vi "test.vi"() -> ()   [LabVIEW 2012]
uses:
  G_SEN.vi
panel:
  out "Array 6":dbl[][](array[numeric])
  out "Array 5":dbl[](array[numeric])
  out "Array 4":i32[](array[numeric])
  out "x*y":dbl[](array[numeric])
  out "Array":dbl[][](array[numeric])
  out "XY Graph 2":cluster{"Y":dbl[], "Y":dbl[]}[](graph)
  out "Array 3":dbl[](array[numeric])
  out "Array 2":cluster{dbl[][]}[](array[cluster])
  out "error out":errorcluster
  out "XY Graph":cluster{"Y":dbl[], "Y":dbl[]}[](graph)
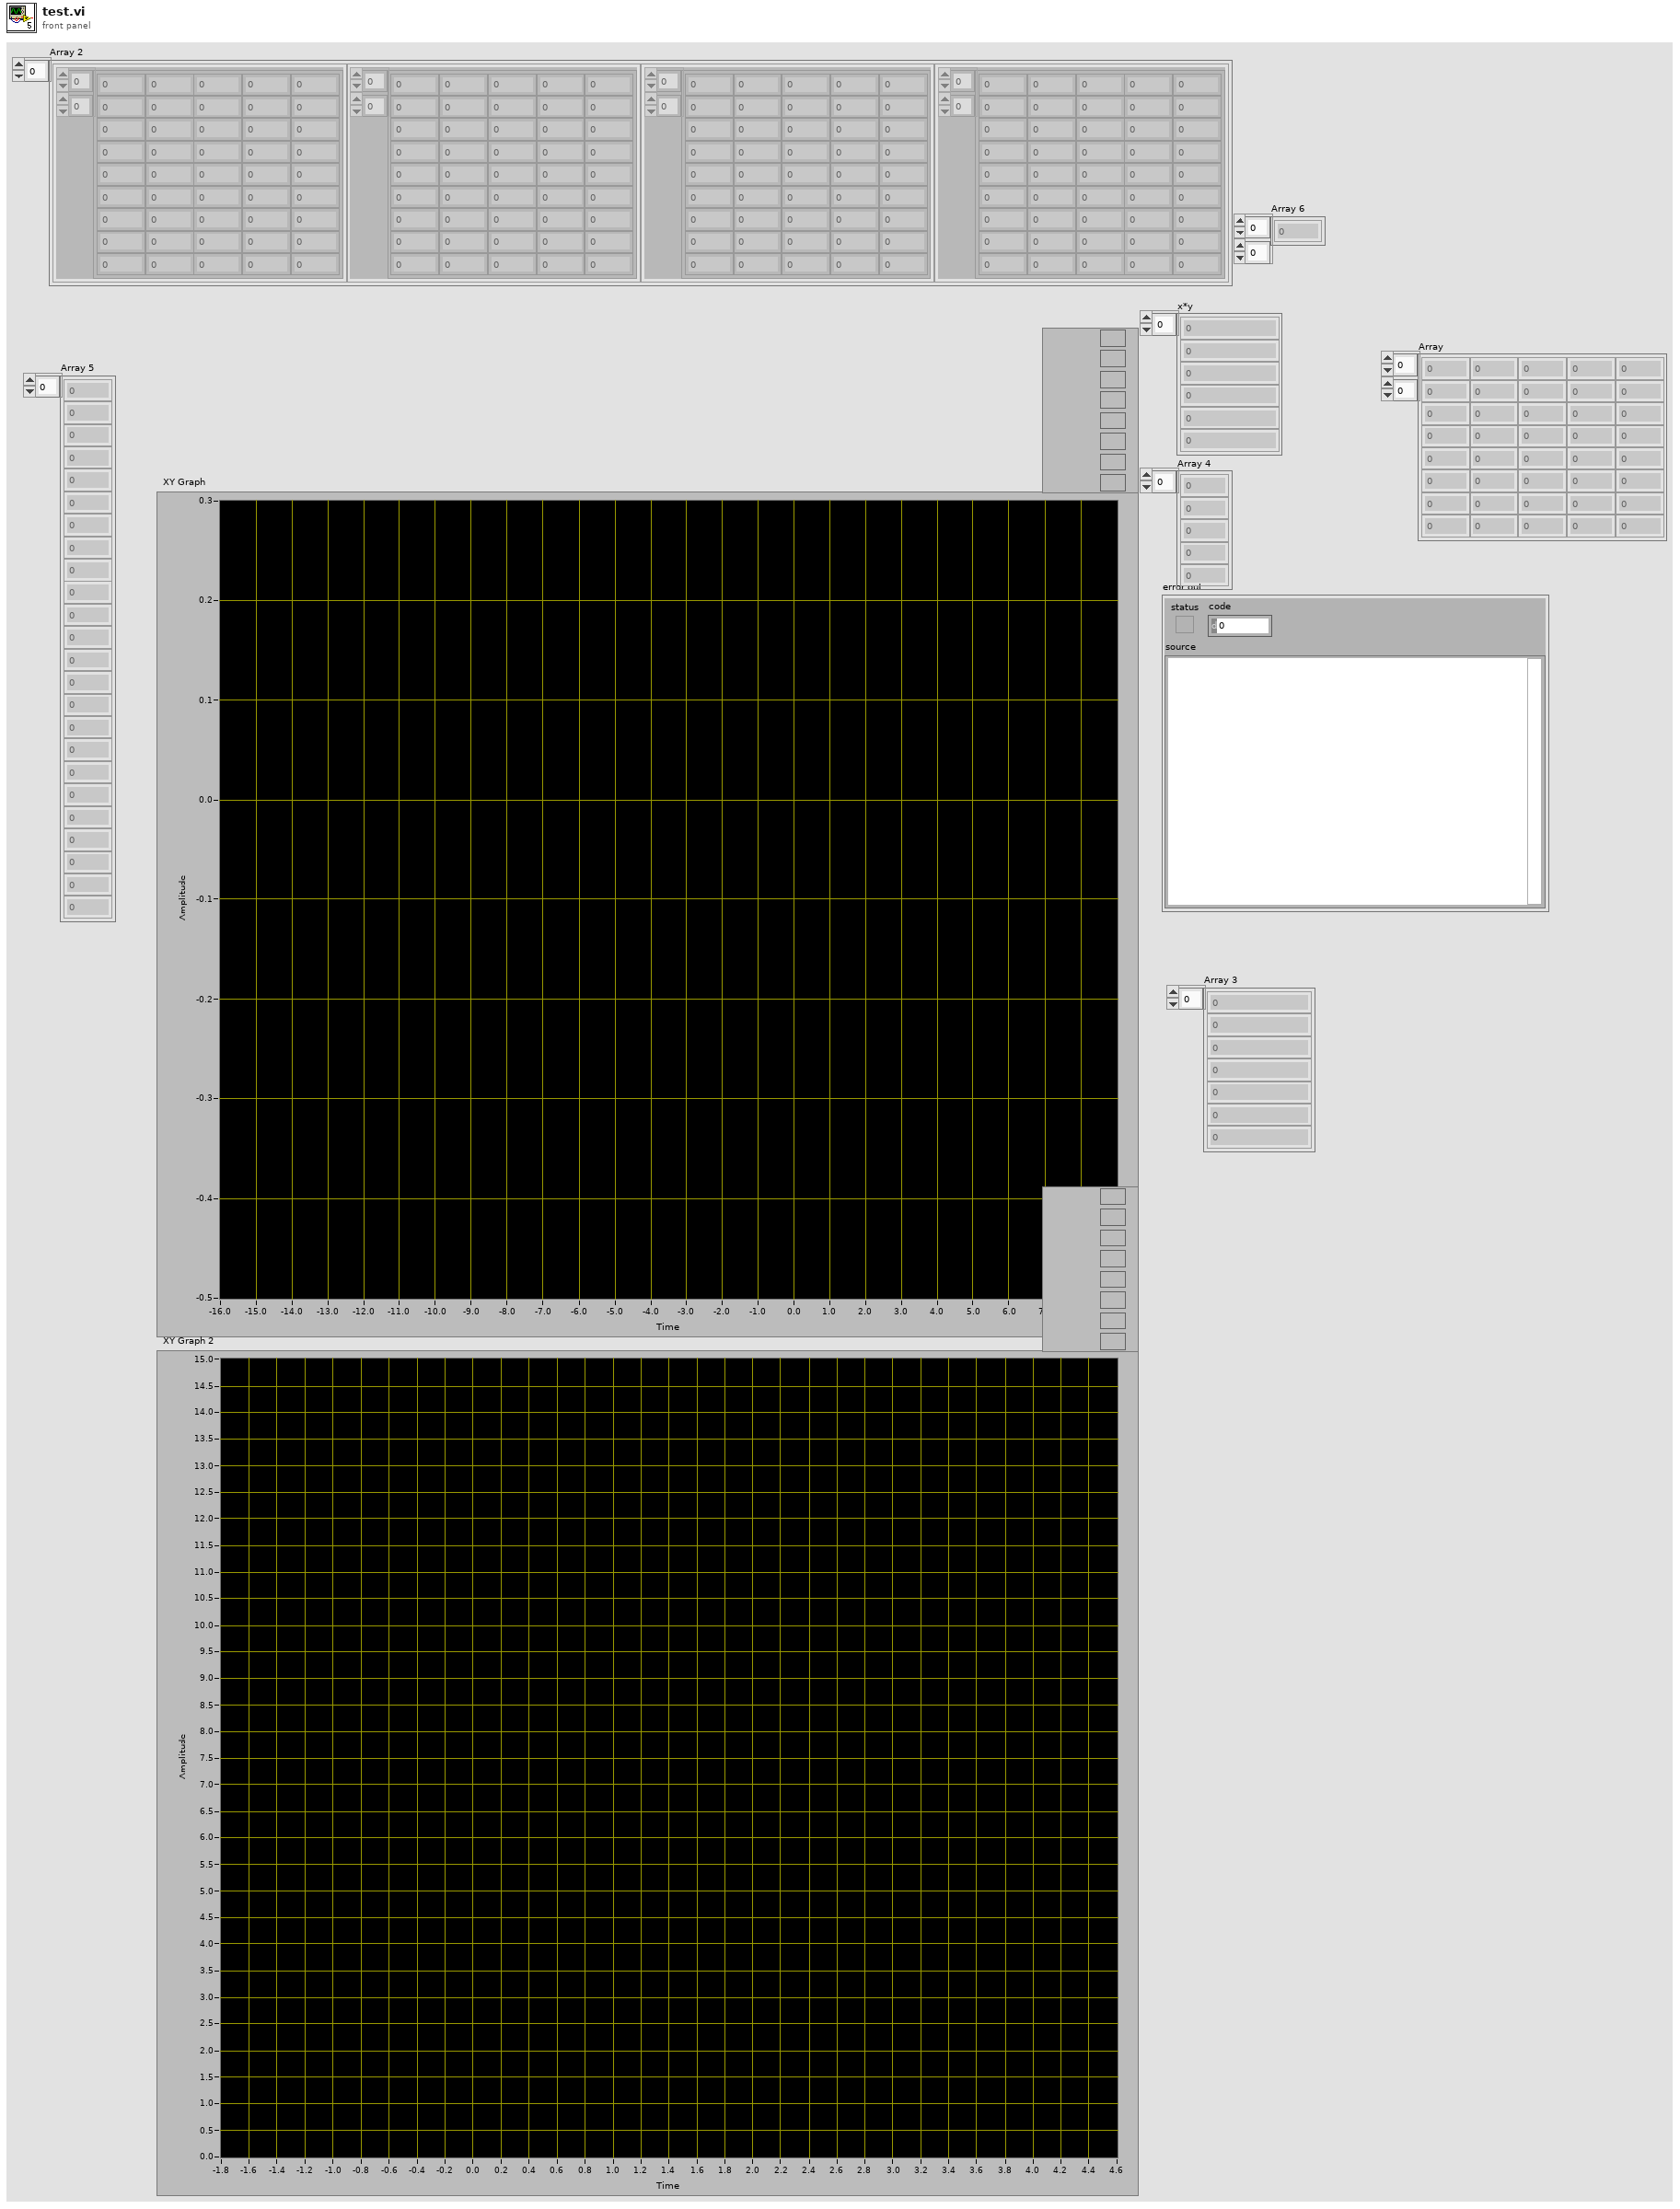
[diagram p1: front panel]
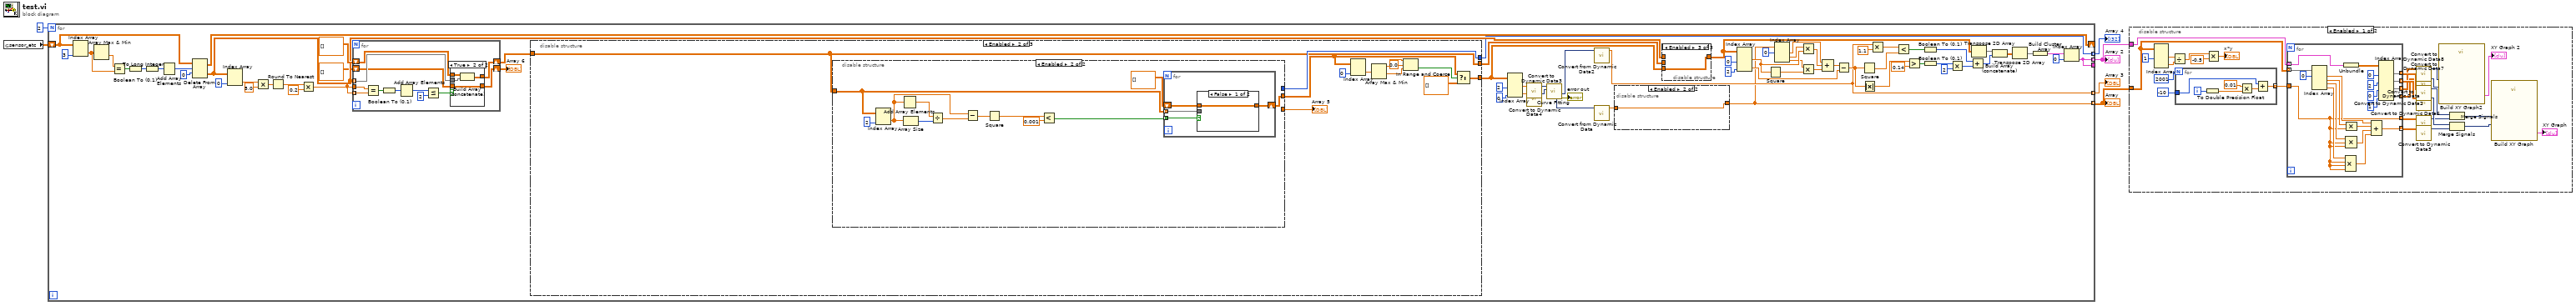
[diagram p0: block diagram]
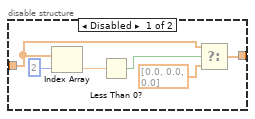
[diagram p3: hidden frame]
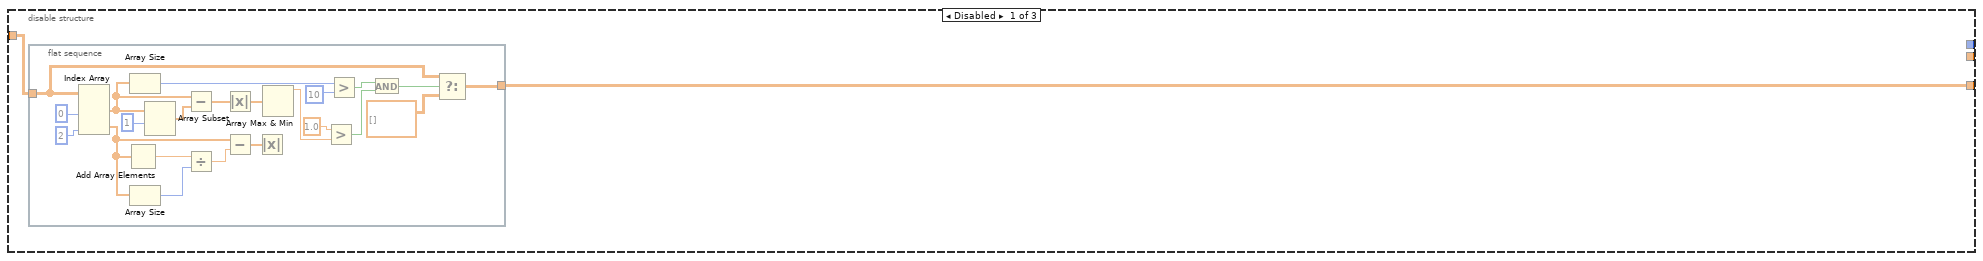
[diagram p4: hidden frame]
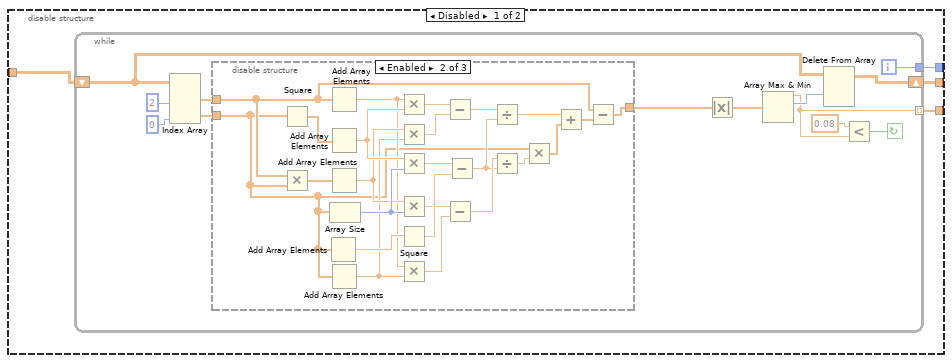
[diagram p5: hidden frame]
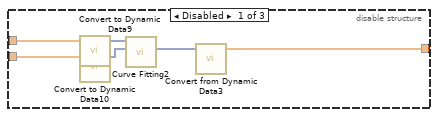
[diagram p6: hidden frame]
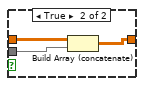
[diagram p8: hidden frame]
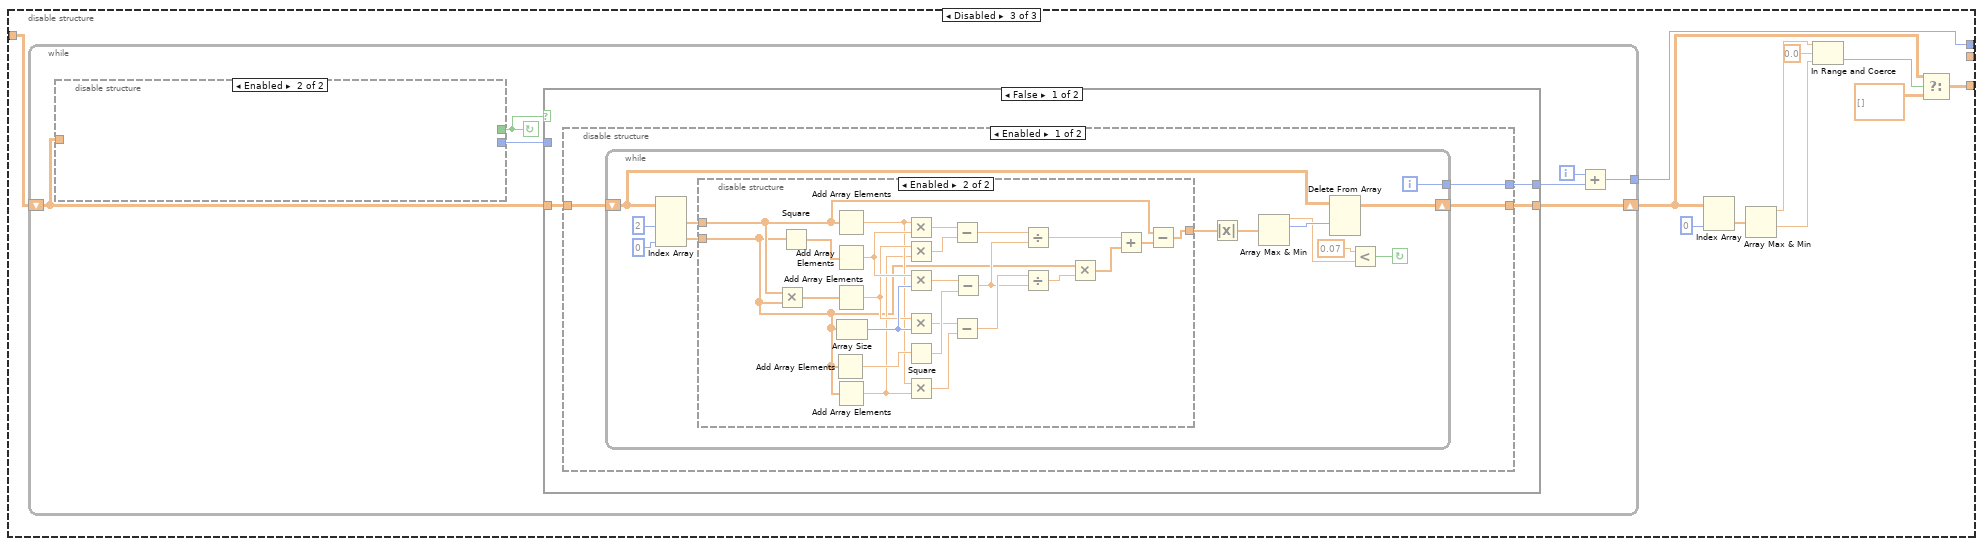
[diagram p9: hidden frame]
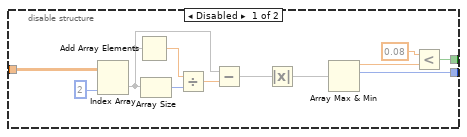
[diagram p10: hidden frame]
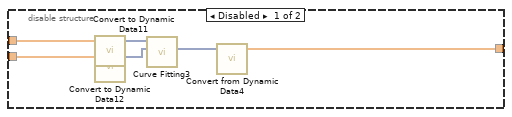
[diagram p11: hidden frame]
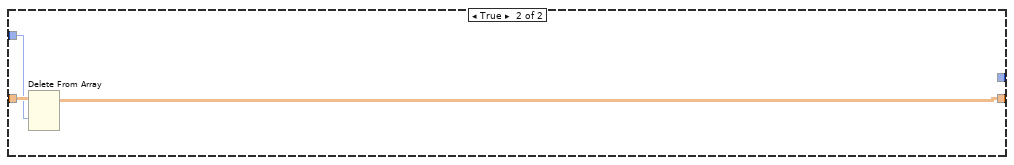
[diagram p13: hidden frame]
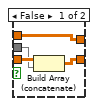
[diagram p16: hidden frame]
diagram:
  n1 = global read "G_SEN.vi" "sensor_etc"() -> (w5:dbl[][])
  n2 = for {
    N: 2 -> [_]
    shift-right: [w66] -> _
    shift-left: w5 -> [w69]
    tunnel: [w14] -> _
    tunnel: [w14] -> w3 mode=indexing
    tunnel: [w13] -> w4 mode=indexing
    tunnel: [w11] -> w2 mode=indexing
    tunnel: [w10] -> w1 mode=indexing
    n3 = Index Array(array=w69, index (col)=3 ("disabled index (col)")) -> (element=w73:dbl[])  [unwired: 1 in]
    n4 = Array Max & Min(array=w73) -> (min value=w74:dbl)  [unwired: 3 out]
    n5 = Equal?(x=w74, y=w73) -> (x = y?=w72:bool[])
    n6 = Boolean To (0,1)(Boolean=w72) -> (0, 1=w71:i16[])
    n7 = To Long Integer(number=w71) -> (32bit integer=w70:i32[])
    n8 = Add Array Elements(numeric array=w70) -> (sum=w68:i32)
    n9 = Delete From Array(array=w69, length=w68, index (row)=0) -> (deleted portion=w18:dbl[][], array with subset deleted=w66:dbl[][])  [unwired: 1 in]
    n10 = Index Array(array=w18, index (col)=0 ("disabled index (col)")) -> (element=w62:dbl[])  [unwired: 1 in]
    n11 = Multiply(x=w62, y=5.0) -> (x*y=w60:dbl[])
    n12 = Round To Nearest(number=w60) -> (nearest integer value=w59:dbl[])
    n13 = Multiply(x=w59, y=0.2) -> (x*y=w57:dbl[])
    n14 = for {
      tunnel: w57 -> [w275] mode=indexing
      tunnel: w57 -> [w283]
      shift-right: [w278] -> w16
      shift-left: dbl[][] [] -> [w279]
      tunnel: w18 -> [w280] mode=indexing
      shift-right: [w272] -> w7
      shift-left: dbl[][] [] -> [w273]
      n15 = Equal?(x=w283, y=w275) -> (x = y?=w282:bool[])
      n16 = Boolean To (0,1)(Boolean=w282) -> (0, 1=w281:i16[])
      n17 = Add Array Elements(numeric array=w281) -> (sum=w277:i16)
      n18 = Less Or Equal?(x=w277, y=i16 2) -> (x <= y?=w274:bool)
      n19 = case shown="True" w274 {
        tunnel: w280 -> [w284 w291]
        tunnel: w279 -> [w287 w290]
        tunnel: [w287 w289] -> w278
        tunnel: w273 -> [w286 w288]
        tunnel: [w285 w288] -> w272
        frame False {
          n20 = Build Array (concatenate)(w286, w284) -> (w285:dbl[][])
        }
        frame True {
          n21 = Build Array (concatenate)(w290, w291) -> (w289:dbl[][])
        }
      }
    }
    "Array 6" <- w7
    n22 = disable-structure shown="Enabled" {
      disable-tunnel: w16 -> [w84 w107 w196]
      disable-tunnel: [w83 w111 w188] -> w15
      disable-tunnel: [_ w109 w186] -> w10
      disable-tunnel: [_ w107 _] -> w9
      frame Disabled {
        n23 = flat-sequence {
          tunnel: w84 -> [w95]
          tunnel: [w94] -> w83
          frame #0 {
            n24 = Index Array(array=w95, index (col) #1=0 ("disabled index (col)"), index (col) #2=2 ("index (col)")) -> (element #1=w102:dbl[], element #2=w86:dbl[])  [unwired: 2 in]
            n25 = Add Array Elements(numeric array=w86) -> (sum=w89:dbl)
            n26 = Array Size(array=w102) -> (size(s)=w101:i32)
            n27 = Array Size(array=w86) -> (size(s)=w88:i32)
            n28 = Array Subset(array=w102, index=1) -> (w103:dbl[])  [unwired: 1 in]
            n29 = Subtract(x=w102, y=w103) -> (x-y=w106:dbl[])
            n30 = Divide(x=w89, y=w88) -> (x/y=w87:dbl)
            n31 = Absolute Value(x=w106) -> (abs(x)=w99:dbl[])
            n32 = Subtract(x=w86, y=w87) -> (x-y=w85:dbl[])
            n33 = Absolute Value(x=w85) -> ()  [unwired: 1 out]
            n34 = Array Max & Min(array=w99) -> (max value=w98:dbl)  [unwired: 3 out]
            n35 = Greater?(x=1.0, y=w98) -> (0:w91:bool)
            n36 = Greater?(x=w101, y=10) -> (0:w92:bool)
            n37 = And(x=w92, y=w91) -> (x .and. y?=w96:bool)
            n38 = Select(t=w95, s=w96, f=dbl[][] []) -> (s? t:f=w94:dbl[][])
          }
        }
      }
      frame Enabled {
        n39 = disable-structure shown="Enabled" {
          disable-tunnel: w107 -> [w122 w171]
          disable-tunnel: [w121 w166] -> w112
          disable-tunnel: [w120 _] -> w109
          disable-tunnel: [w119 _] -> w108
          frame Disabled {
            n40 = while {
              shift-right: [w130] -> w121
              shift-left: w122 -> [w131]
              tunnel: [w127] -> w120
              tunnel: [w123] -> w119 mode=indexing
              i -> [w127]
              stop <- w128 continue-if-true
              n41 = Index Array(array=w131, index (col) #1=2 ("disabled index (col)"), index (col) #2=0 ("index (col)")) -> (element #1=w135:dbl[], element #2=w124:dbl[])  [unwired: 2 in]
              n42 = disable-structure shown="Enabled" {
                disable-tunnel: w135 -> [w141 w147 _]
                disable-tunnel: [w137 w146 _] -> w126
                disable-tunnel: w124 -> [w136 w144 _]
                frame Disabled {
                  n43 = call "Convert to Dynamic Data9"("Array"=w141) -> ("Dynamic Data Type"=w139:dynamicdata)  [unwired: 3 in]
                  n44 = call "Convert to Dynamic Data10"("Array"=w136) -> ("Dynamic Data Type"=w140:dynamicdata)  [unwired: 3 in]
                  n45 = call "Curve Fitting2"("Locations"=w140, "Signals"=w139) -> ("residual"=w138:dynamicdata)  [unwired: 5 in, 4 out]
                  n46 = call "Convert from Dynamic Data3"("Dynamic Data Type"=w138) -> ("Array"=w137:dbl[])  [unwired: 3 in]
                }
                frame Enabled {
                  n47 = Square(x=w144) -> (x^2=w165:dbl[])
                  n48 = Multiply(x=w147, y=w144) -> (x*y=w161:dbl[])
                  n49 = Add Array Elements(numeric array=w144) -> (sum=w164:dbl)
                  n50 = Add Array Elements(numeric array=w147) -> (sum=w153:dbl)
                  n51 = Add Array Elements(numeric array=w165) -> (sum=w162:dbl)
                  n52 = Add Array Elements(numeric array=w161) -> (sum=w155:dbl)
                  n53 = Add Array Elements(numeric array=w144) -> (sum=w152:dbl)
                  n54 = Array Size(array=w144) -> (size(s)=w156:i32)
                  n55 = Multiply(x=w153, y=w162) -> (x*y=w159:dbl)
                  n56 = Multiply(x=w155, y=w152) -> (x*y=w160:dbl)
                  n57 = Multiply(x=w162, y=w156) -> (x*y=w157:dbl)
                  n58 = Multiply(x=w155, y=w156) -> (x*y=w154:dbl)
                  n59 = Square(x=w164) -> (x^2=w163:dbl)
                  n60 = Multiply(x=w153, y=w152) -> (x*y=w151:dbl)
                  n61 = Subtract(x=w159, y=w160) -> (x-y=w158:dbl)
                  n62 = Subtract(x=w154, y=w151) -> (x-y=w150:dbl)
                  n63 = Subtract(x=w157, y=w163) -> (x-y=w149:dbl)
                  n64 = Divide(x=w158, y=w149) -> (x/y=w145:dbl)
                  n65 = Divide(x=w150, y=w149) -> (x/y=w143:dbl)
                  n66 = Multiply(x=w144, y=w143) -> (x*y=w142:dbl[])
                  n67 = Add(x=w145, y=w142) -> (x+y=w148:dbl[])
                  n68 = Subtract(x=w147, y=w148) -> (x-y=w146:dbl[])
                }
                frame Disabled {
                }
              }
              n69 = Absolute Value(x=w126) -> (abs(x)=w125:dbl[])
              n70 = Array Max & Min(array=w125) -> (max value=w123:dbl, max index (indices)=w132:i32)  [unwired: 2 out]
              n71 = Delete From Array(array=w131, index (row)=w132) -> (array with subset deleted=w130:dbl[][])  [unwired: 2 in, 1 out]
              n72 = Less?(x=0.08, y=w123) -> (x < y?=w128:bool)
            }
          }
          frame Enabled {
            n73 = Index Array(array=w171, index (col)=2 ("disabled index (col)")) -> (element=w173:dbl[])  [unwired: 1 in]
            n74 = Add Array Elements(numeric array=w173) -> (sum=w176:dbl)
            n75 = Array Size(array=w173) -> (size(s)=w172:i32)
            n76 = Divide(x=w176, y=w172) -> (x/y=w175:dbl)
            n77 = Subtract(x=w173, y=w175) -> (x-y=w174:dbl[])
            n78 = Square(x=w174) -> (x^2=w170:dbl[])
            n79 = Less?(x=w170, y=0.001) -> (x < y?=w168:bool[])
            n80 = for {
              tunnel: w171 -> [w180] mode=indexing
              tunnel: w168 -> [w181] mode=indexing
              shift-right: [w178] -> w166
              shift-left: dbl[][] [] -> [w179]
              n81 = case shown="False" w181 {
                tunnel: w180 -> [_ w185]
                tunnel: w179 -> [w182 w184]
                tunnel: [w182 w183] -> w178
                frame False {
                }
                frame True {
                  n82 = Build Array (concatenate)(w184, w185) -> (w183:dbl[][])
                }
              }
            }
          }
        }
        "Array 5" <- w108
        n83 = Index Array(array=w112, index (col)=0 ("disabled index (col)")) -> (element=w117:dbl[])  [unwired: 1 in]
        n84 = Array Max & Min(array=w117) -> (max value=w116:dbl, min value=w115:dbl)  [unwired: 2 out]
        n85 = In Range and Coerce(upper limit=w116, x=0.0, lower limit=w115) -> (In Range?=w113:bool)  [unwired: 1 out]
        n86 = Select(t=w112, s=w113, f=dbl[][] []) -> (s? t:f=w111:dbl[][])
      }
      frame Disabled {
        n87 = while {
          shift-right: [w201] -> w189
          shift-left: w196 -> [w202]
          tunnel: [w197] -> w186
          i -> [w199]
          stop <- w203 continue-if-true
          n88 = disable-structure shown="Enabled" {
            disable-tunnel: [w207 _] -> w203
            disable-tunnel: w202 -> [w206 _]
            disable-tunnel: [w205 _] -> w200
            frame Disabled {
              n89 = Index Array(array=w206, index (col)=2 ("disabled index (col)")) -> (element=w211:dbl[])  [unwired: 1 in]
              n90 = Add Array Elements(numeric array=w211) -> (sum=w214:dbl)
              n91 = Array Size(array=w211) -> (size(s)=w213:i32)
              n92 = Divide(x=w214, y=w213) -> (x/y=w212:dbl)
              n93 = Subtract(x=w211, y=w212) -> (x-y=w210:dbl[])
              n94 = Absolute Value(x=w210) -> (abs(x)=w209:dbl[])
              n95 = Array Max & Min(array=w209) -> (max value=w208:dbl, max index (indices)=w205:i32)  [unwired: 2 out]
              n96 = Less?(x=0.08, y=w208) -> (x < y?=w207:bool)
            }
            frame Enabled {
            }
          }
          n97 = case shown="False" w203 {
            tunnel: w202 -> [w218 w268]
            tunnel: [w217 w267] -> w201
            tunnel: w200 -> [_ w266]
            tunnel: [w216 _] -> w198
            frame False {
              n98 = disable-structure shown="Enabled" {
                disable-tunnel: w218 -> [w221 w265]
                disable-tunnel: [w220 w265] -> w217
                disable-tunnel: [w219 _] -> w216
                frame Enabled {
                  n99 = while {
                    shift-right: [w229] -> w220
                    shift-left: w221 -> [w230]
                    tunnel: [w225] -> w219
                    i -> [w225]
                    stop <- w226 continue-if-true
                    n100 = Index Array(array=w230, index (col) #1=2 ("disabled index (col)"), index (col) #2=0 ("index (col)")) -> (element #1=w234:dbl[], element #2=w222:dbl[])  [unwired: 2 in]
                    n101 = disable-structure shown="Enabled" {
                      disable-tunnel: w234 -> [w240 w246]
                      disable-tunnel: [w236 w245] -> w224
                      disable-tunnel: w222 -> [w235 w243]
                      frame Disabled {
                        n102 = call "Convert to Dynamic Data11"("Array"=w240) -> ("Dynamic Data Type"=w238:dynamicdata)  [unwired: 3 in]
                        n103 = call "Convert to Dynamic Data12"("Array"=w235) -> ("Dynamic Data Type"=w239:dynamicdata)  [unwired: 3 in]
                        n104 = call "Curve Fitting3"("Locations"=w239, "Signals"=w238) -> ("residual"=w237:dynamicdata)  [unwired: 5 in, 4 out]
                        n105 = call "Convert from Dynamic Data4"("Dynamic Data Type"=w237) -> ("Array"=w236:dbl[])  [unwired: 3 in]
                      }
                      frame Enabled {
                        n106 = Multiply(x=w246, y=w243) -> (x*y=w260:dbl[])
                        n107 = Square(x=w243) -> (x^2=w264:dbl[])
                        n108 = Add Array Elements(numeric array=w243) -> (sum=w263:dbl)
                        n109 = Add Array Elements(numeric array=w246) -> (sum=w252:dbl)
                        n110 = Add Array Elements(numeric array=w264) -> (sum=w261:dbl)
                        n111 = Add Array Elements(numeric array=w260) -> (sum=w254:dbl)
                        n112 = Add Array Elements(numeric array=w243) -> (sum=w251:dbl)
                        n113 = Array Size(array=w243) -> (size(s)=w255:i32)
                        n114 = Multiply(x=w252, y=w261) -> (x*y=w258:dbl)
                        n115 = Multiply(x=w254, y=w251) -> (x*y=w259:dbl)
                        n116 = Multiply(x=w261, y=w255) -> (x*y=w256:dbl)
                        n117 = Multiply(x=w254, y=w255) -> (x*y=w253:dbl)
                        n118 = Square(x=w263) -> (x^2=w262:dbl)
                        n119 = Multiply(x=w252, y=w251) -> (x*y=w250:dbl)
                        n120 = Subtract(x=w258, y=w259) -> (x-y=w257:dbl)
                        n121 = Subtract(x=w253, y=w250) -> (x-y=w249:dbl)
                        n122 = Subtract(x=w256, y=w262) -> (x-y=w248:dbl)
                        n123 = Divide(x=w257, y=w248) -> (x/y=w244:dbl)
                        n124 = Divide(x=w249, y=w248) -> (x/y=w242:dbl)
                        n125 = Multiply(x=w243, y=w242) -> (x*y=w241:dbl[])
                        n126 = Add(x=w244, y=w241) -> (x+y=w247:dbl[])
                        n127 = Subtract(x=w246, y=w247) -> (x-y=w245:dbl[])
                      }
                    }
                    n128 = Absolute Value(x=w224) -> (abs(x)=w223:dbl[])
                    n129 = Array Max & Min(array=w223) -> (max value=w227:dbl, max index (indices)=w231:i32)  [unwired: 2 out]
                    n130 = Delete From Array(array=w230, index (row)=w231) -> (array with subset deleted=w229:dbl[][])  [unwired: 2 in, 1 out]
                    n131 = Less?(x=0.07, y=w227) -> (x < y?=w226:bool)
                  }
                }
                frame Disabled {
                }
              }
            }
            frame True {
              n132 = Delete From Array(array=w268, index (row)=w266) -> (array with subset deleted=w267:dbl[][])  [unwired: 2 in, 1 out]
            }
          }
          n133 = Add(x=w199, y=w198) -> (x+y=w197:i32)
        }
        n134 = Index Array(array=w189, index (col)=0 ("disabled index (col)")) -> (element=w194:dbl[])  [unwired: 1 in]
        n135 = Array Max & Min(array=w194) -> (max value=w193:dbl, min value=w192:dbl)  [unwired: 2 out]
        n136 = In Range and Coerce(upper limit=w193, x=0.0, lower limit=w192) -> (In Range?=w190:bool)  [unwired: 1 out]
        n137 = Select(t=w189, s=w190, f=dbl[][] []) -> (s? t:f=w188:dbl[][])
      }
    }
    n138 = Index Array(array=w15, index (col) #1=2 ("disabled index (col)"), index (col) #2=0 ("index (col)")) -> (element #1=w48:dbl[], element #2=w52:dbl[])  [unwired: 2 in]
    n139 = call "Convert to Dynamic Data3"("Array"=w48) -> ("Dynamic Data Type"=w53:dynamicdata)  [unwired: 3 in]
    n140 = call "Convert to Dynamic Data4"("Array"=w52) -> ("Dynamic Data Type"=w51:dynamicdata)  [unwired: 3 in]
    n141 = call "Curve Fitting"("Locations"=w51, "Signals"=w53) -> ("error out"=→"error out":errorcluster, "mean squared error"=w49:dynamicdata, "polynomial coefficients"=w50:dynamicdata)  [unwired: 5 in, 2 out]
    n142 = call "Convert from Dynamic Data2"("Dynamic Data Type"=w49) -> ("Scalar"=w13:dbl)  [unwired: 3 in]
    n143 = call "Convert from Dynamic Data"("Dynamic Data Type"=w50) -> ("Array"=w12:dbl[])  [unwired: 3 in]
    n144 = disable-structure shown="Enabled" {
      disable-tunnel: w12 -> [w78 w82]
      disable-tunnel: [w77 w82] -> w11
      frame Disabled {
        n145 = Index Array(array=w78, index=2) -> (element=w80:dbl)
        n146 = Less Than 0?(x=w80) -> (x < 0?=w79:bool)
        n147 = Select(t=w78, s=w79, f=dbl[] [0.0, 0.0, 0.0]) -> (s? t:f=w77:dbl[])
      }
      frame Enabled {
      }
    }
    n148 = disable-structure shown="Enabled" {
      disable-tunnel: w18 -> [w269 _ _]
      disable-tunnel: [w269 w270 w271] -> w17
      disable-tunnel: w15 -> [_ _ w271]
      disable-tunnel: w9 -> [_ w270 _]
      frame Disabled {
      }
      frame Disabled {
      }
      frame Enabled {
      }
    }
    n149 = Index Array(array=w17, index (col) #1=0 ("disabled index (col)"), index (col) #2=2 ("index (col)")) -> (element #1=w44:dbl[], element #2=w36:dbl[])  [unwired: 2 in]
    n150 = Square(x=w44) -> (x^2=w42:dbl[])
    n151 = Index Array(array=w11, index #1=0 ("index")) -> (element #1=w41:dbl, element #2=w45:dbl, element #3=w43:dbl)  [unwired: 2 in]
    n152 = Multiply(x=w45, y=w44) -> (x*y=w40:dbl[])
    n153 = Multiply(x=w43, y=w42) -> (x*y=w39:dbl[])
    n154 = Compound Arithmetic op=ADD(w41, w40, w39) -> (w37:dbl[])
    n155 = Subtract(x=w37, y=w36) -> (x-y=w28:dbl[])
    n156 = Square(x=w28) -> (x^2=w33:dbl[])
    n157 = Absolute Value(x=w28) -> (abs(x)=w27:dbl[])
    n158 = Multiply(x=w13, y=1.1) -> (x*y=w34:dbl)
    n159 = Less?(x=w34, y=w33) -> (x < y?=w31:bool[])
    n160 = Greater?(x=w27, y=0.14) -> (0:w25:bool[])
    n161 = Boolean To (0,1)(Boolean=w31) -> (0, 1=w24:i16[])
    n162 = Boolean To (0,1)(Boolean=w25) -> (0, 1=w22:i16[])
    n163 = Multiply(x=w22, y=i16 2) -> (x*y=w20:i16[])
    n164 = Add(x=w24, y=w20) -> (x+y=w23:i16[])
    n165 = Transpose 2D Array(2D array=w17) -> (transposed array=w32:dbl[][])
    n166 = Build Array (concatenate)(w32, w23) -> (w30:dbl[][])
    n167 = Transpose 2D Array(2D array=w30) -> (transposed array=w29:dbl[][])
    n168 = Build Cluster Array(w29) -> (w65:cluster{dbl[][]}[])
    n169 = Index Array(array=w65, index=0) -> (element=w14:cluster{dbl[][]})
  }
  "Array 2" <- w3
  "Array 3" <- w4
  "Array" <- w2
  "Array 4" <- w1
  n170 = disable-structure shown="Enabled" {
    disable-tunnel: w3 -> [w305 _]
    disable-tunnel: w2 -> [w298 _]
    frame Enabled {
      n171 = Index Array(array=w298, index (col) #1=1 ("disabled index (col)")) -> (element #1=w296:dbl[], element #2=w295:dbl[])  [unwired: 3 in]
      n172 = Divide(x=w296, y=w295) -> (x/y=w294:dbl[])
      n173 = for {
        N: 2001 -> [_]
        tunnel: -10 -> [w321]
        tunnel: [w319] -> w315 mode=indexing
        i -> [w324]
        n174 = To Double Precision Float(number=w324) -> (double precision float=w323:dbl)
        n175 = Multiply(x=0.01, y=w323) -> (x*y=w320:dbl)
        n176 = Add(x=w321, y=w320) -> (x+y=w319:dbl)
      }
      n177 = Multiply(x=w294, y=-0.5) -> (x*y=→"x*y":dbl[])
      n178 = for {
        tunnel: w305 -> [w345] mode=indexing
        tunnel: [w340] -> w314 mode=indexing
        tunnel: [w339] -> w313 mode=indexing
        tunnel: w315 -> [w326]
        tunnel: w298 -> [w338] mode=indexing
        tunnel: [w326] -> w307 mode=indexing
        tunnel: [w331] -> w310 mode=indexing
        tunnel: [w329] -> w303 mode=indexing
        tunnel: [w328] -> w300 mode=indexing
        n179 = Index Array(array=w338, index #1=0 ("index")) -> (element #1=w334:dbl, element #2=w336:dbl, element #3=w335:dbl, element #4=w327:dbl)  [unwired: 3 in]
        n180 = Unbundle(w345) -> (w342:dbl[][])
        n181 = Compound Arithmetic op=MULTIPLY(w327, w326, w326, w326) -> (w325:dbl[])
        n182 = Compound Arithmetic op=MULTIPLY(w335, w326, w326) -> (w332:dbl[])
        n183 = Compound Arithmetic op=MULTIPLY(w336, w326) -> (w333:dbl[])
        n184 = Compound Arithmetic op=ADD(w334, w333, w332, w325) -> (w331:dbl[])
        n185 = Index Array(array=w342, index (col) #1=0 ("disabled index (col)"), index (col) #2=2 ("index (col)"), index (col) #3=0 ("index (col)"), index (col) #4=1 ("index (col)")) -> (element #1=w340:dbl[], element #2=w339:dbl[], element #3=w328:dbl[], element #4=w329:dbl[])  [unwired: 4 in]
      }
      n186 = call "Convert to Dynamic Data8"("2D Array"=w300) -> ("Dynamic Data Type"=w299:dynamicdata)  [unwired: 3 in]
      n187 = call "Convert to Dynamic Data7"("2D Array"=w303) -> ("Dynamic Data Type"=w302:dynamicdata)  [unwired: 3 in]
      n188 = call "Convert to Dynamic Data"("2D Array"=w314) -> ("Dynamic Data Type"=w304:dynamicdata)  [unwired: 3 in]
      n189 = call "Convert to Dynamic Data2"("2D Array"=w313) -> ("Dynamic Data Type"=w312:dynamicdata)  [unwired: 3 in]
      n190 = call "Convert to Dynamic Data6"("2D Array"=w307) -> ("Dynamic Data Type"=w306:dynamicdata)  [unwired: 3 in]
      n191 = call "Convert to Dynamic Data5"("2D Array"=w310) -> ("Dynamic Data Type"=w309:dynamicdata)  [unwired: 3 in]
      n192 = call "Build XY Graph2"("Y Input"=w302, "X Input"=w299) -> ("XY Graph"=→"XY Graph 2":cluster{"Y":dbl[], "Y":dbl[]}[])  [unwired: 3 in, 6 out]
      n193 = Merge Signals(w304, w306) -> (w308:dynamicdata)
      n194 = Merge Signals(w312, w309) -> (w311:dynamicdata)
      n195 = call "Build XY Graph"("Y Input"=w311, "X Input"=w308) -> ("XY Graph"=→"XY Graph":cluster{"Y":dbl[], "Y":dbl[]}[])  [unwired: 3 in, 6 out]
    }
    frame Disabled {
    }
  }
